vi "TSP Plot_05_15_18_AZ.vi"(8 "Transport Graph Properties":T1={"Transport Line Size"=0, "Transport Line Color"=16774656} {"Transport Line Size" items=["Extra Small", "Small", "Medium", "Large", "Extra Large"]}, 9 "No Transport File":path=path "\\\\acad1\\physics/Jurchescu-group/JW-PD/Mega Awesome/No Transport File.txt", 10 "Transport Folder":path) -> (1 "Transport":cluster{ext[], ext[]}[](graph), 2 "Transport File":path, 3 "Transport Name":string)   [LabVIEW 2015]
uses:
  <vilib>/Utility/file.llb/Read From Spreadsheet File (string).vi
panel:
  in  "stop":bool
  in  "Numeric":i64
  in  "default (0 dbl)":ext format="%.2e"
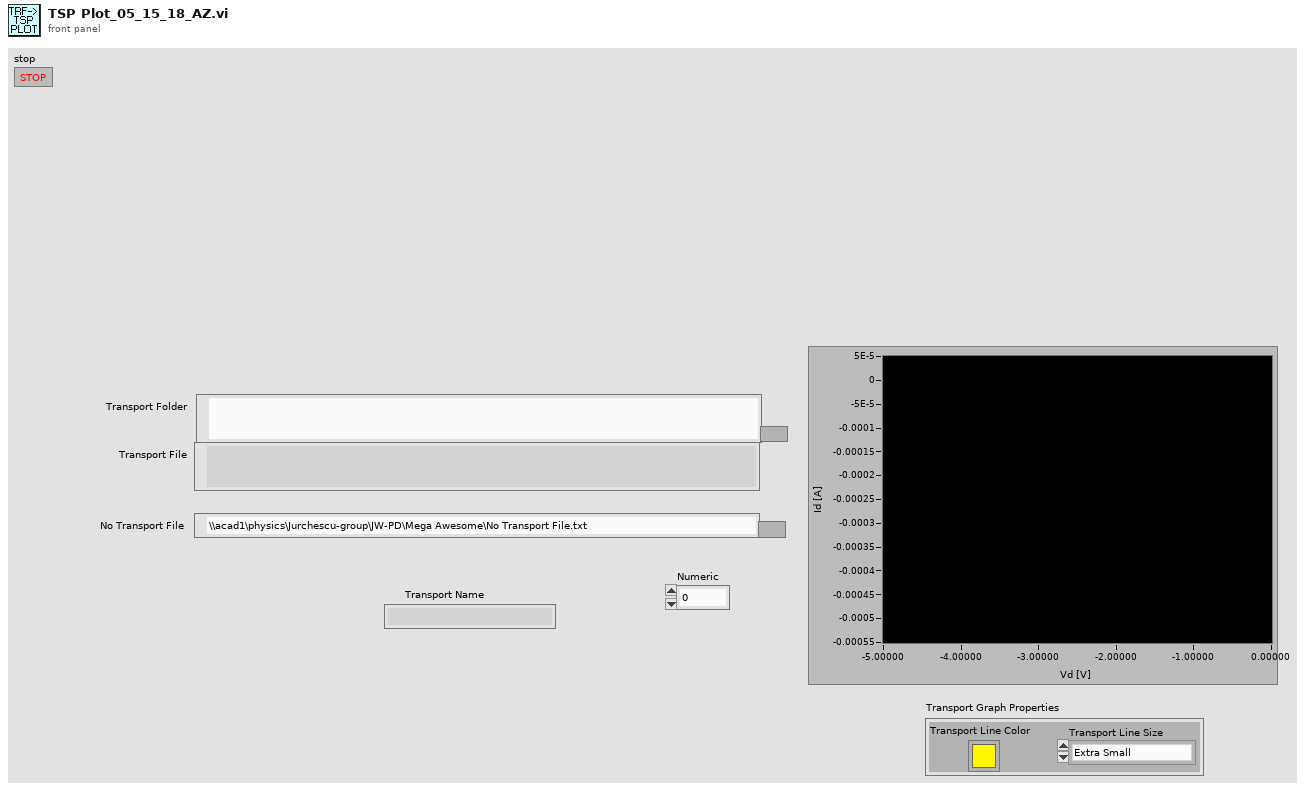
[diagram p1: front panel]
types:
  T1 = cluster{"Transport Line Size":u16, "Transport Line Color":u32}
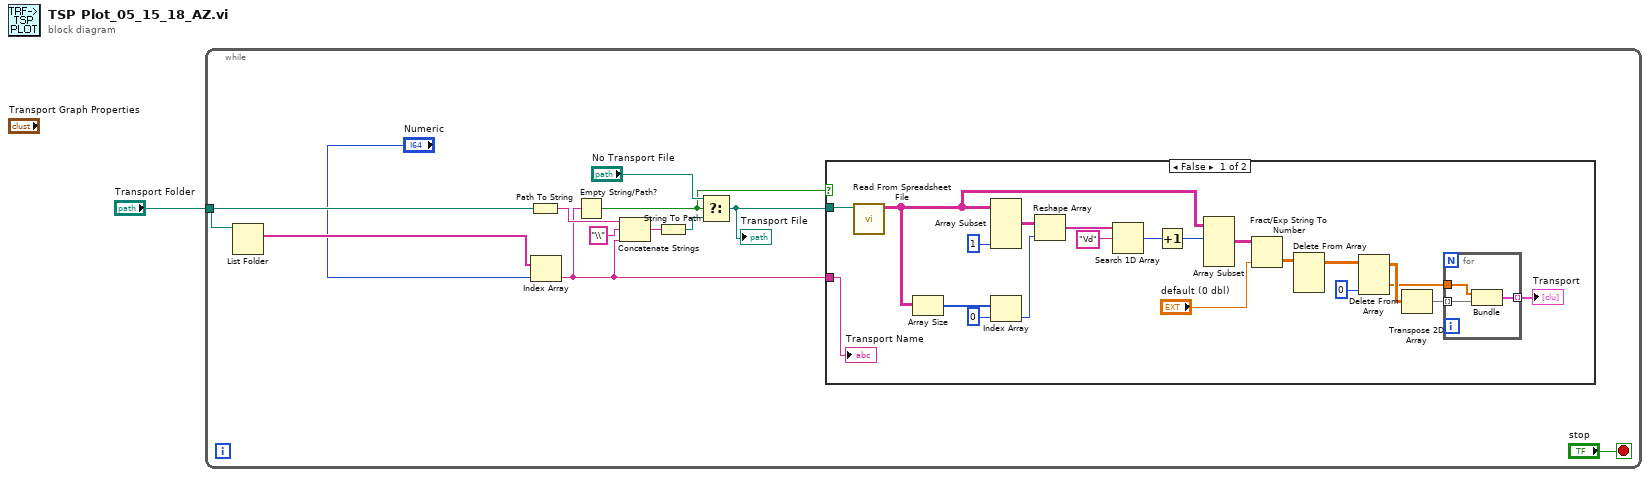
[diagram p0: block diagram]
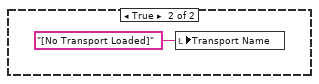
[diagram p2: hidden frame]
diagram:
  n1 = while {
    tunnel: "Transport Folder" -> [w13]
    stop <- "stop" stop-if-true
    n2 = List Folder(path=w13) -> (filenames=w12:string[])  [unwired: 3 in, 3 out]
    n3 = Path To String(path=w13) -> (string=w9:string)
    n4 = Index Array(array=w12, index="Numeric") -> (element=w6:string)
    n5 = Empty String/Path?(string/path=w6) -> (empty?=w4:bool)
    n6 = Concatenate Strings(w9, "\\", w6) -> (w10:string)
    n7 = String To Path(string=w10) -> (path=w7:path)
    n8 = Select(t="No Transport File", s=w4, f=w7) -> (s? t:f=w8:path)
    "Transport File" <- w8
    n9 = case shown="False" w4 {
      tunnel: w8 -> [w34 _]
      tunnel: w6 -> [w14 _]
      frame False {
        n10 = call-poly <vilib>:"Read From Spreadsheet File.vi"("file path (dialog if empty)"=w34) -> ("all rows"=w27:string[][])  [unwired: 6 in, 4 out]
        n11 = Array Size(array=w27) -> (size(s)=w33:i32[])
        n12 = Array Subset(array=w27, length (col)=1) -> (w29:string[][])  [unwired: 3 in]
        n13 = Index Array(array=w33, index=0) -> (element=w22:i32)
        n14 = Reshape Array(w29, w22) -> (w28:string[])
        n15 = Search 1D Array(1D array=w28, element="Vd") -> (index of element=w26:i32)  [unwired: 1 in]
        n16 = Increment(x=w26) -> (x+1=w25:i32)
        n17 = Array Subset(array=w27, index (row)=w25) -> (w23:string[][])  [unwired: 3 in]
        n18 = Fract/Exp String To Number(string=w23, default (0 dbl)="default (0 dbl)") -> (number=w17:ext[][])  [unwired: 2 in, 1 out]
        n19 = Delete From Array(array=w17) -> (array with subset deleted=w16:ext[][])  [unwired: 3 in, 1 out]
        n20 = Delete From Array(array=w16, index (col)=0 ("Deaktivierter Index (Spalte)")) -> (deleted portion=w19:ext[], array with subset deleted=w20:ext[][])  [unwired: 2 in]
        n21 = Transpose 2D Array(2D array=w20) -> (transposed array=w21:ext[][])
        n22 = for {
          tunnel: w19 -> [w36]
          tunnel: w21 -> [w37] mode=indexing
          tunnel: [w35] -> w15 mode=indexing
          n23 = Bundle(w36, w37) -> (w35:cluster{ext[], ext[]})  [unwired: 1 in]
        }
        "Transport" <- w15
        "Transport Name" <- w14
      }
      frame True {
        n24 = local write "Transport Name"("[No Transport Loaded]") -> ()
      }
    }
  }
